vi "Move Point.vi"(10 "Direction":T2=enum."Center", 11 "Start Point":T1) -> (3 "New Point":T1)   [LabVIEW 2020]
uses:
  Cluster _Point Location.ctl
  ENUM_Location Direction.ctl
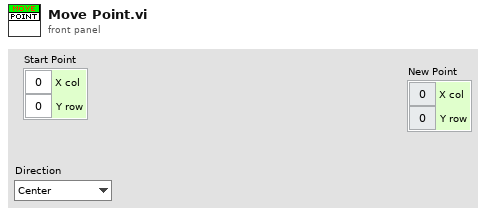
[diagram p1: front panel]
types:
  T1 = typedef "Cluster _Point Location.ctl" = cluster{"X col":i32, "Y row":i32}
  T2 = typedef "ENUM_Location Direction.ctl" = enum16{"North", "North-East", "East", "South-East", "South", "South-West", "West", "North-West", "Center"}
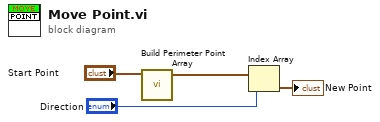
[diagram p0: block diagram]
diagram:
  n1 = call "Build Perimeter Point Array.vi"("Start Point"="Start Point") -> ("No Center Out"=w3:T1[])  [unwired: 7 in, 3 out]
  n2 = Index Array(array=w3, index="Direction") -> (element=→"New Point":T1)
